vi "Remove NaNs.vi"(1 "Array in":dbl[](array[numeric])) -> (0 "Array out":dbl[](array[numeric]))   [LabVIEW 2020, in "Retrieve and Visualize.lvclass"]
uses:
  Retrieve and Visualize.lvclass
  Retrieve and Visualize.lvclass/Retrieve and Visualize.ctl
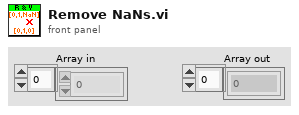
[diagram p1: front panel]
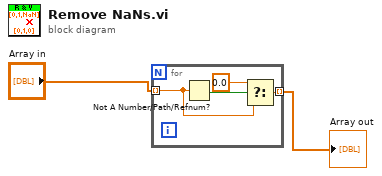
[diagram p0: block diagram]
diagram:
  n1 = for {
    tunnel: [w6] -> w2 mode=indexing
    tunnel: "Array in" -> [w3] mode=indexing
    n2 = Not A Number/Path/Refnum?(number/path/refnum=w3) -> (NaN/Path/Refnum?=w5:bool)
    n3 = Select(t=0.0, s=w5, f=w3) -> (s? t:f=w6:dbl)
  }
  "Array out" <- w2
